vi "Update Speed.vi"(2 "error in (no error)":errorcluster, 3 "Time Since Last Update":dbl, 4 "Car.lvclass":refnum<class "Car.lvclass">) -> (0 "error out":errorcluster, 1 "Car.lvclass 2":refnum<class "Car.lvclass">)   [LabVIEW 2015, in "Car.lvclass"]
uses:
  Car.lvclass
  Car.lvclass/Car.ctl
panel:
  in  "Acceleration Rate":dbl=20.0
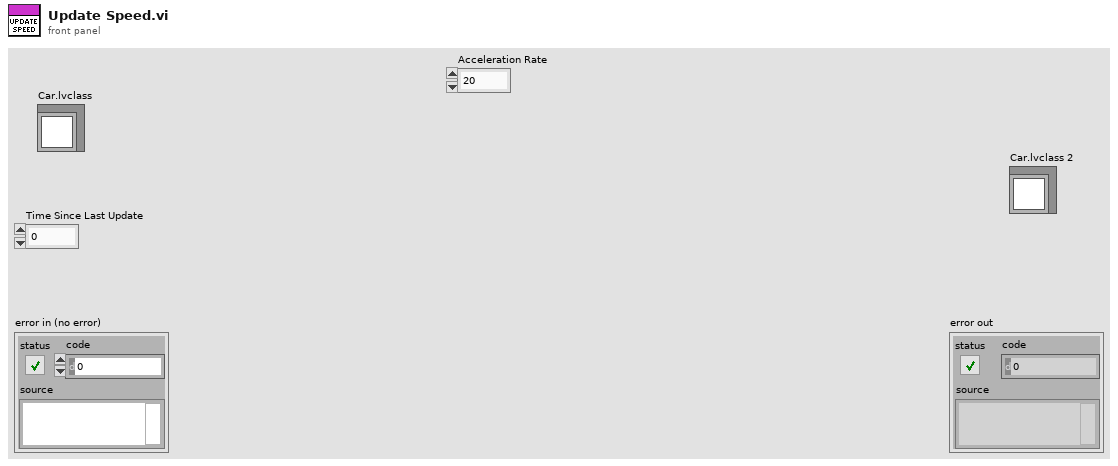
[diagram p1: front panel]
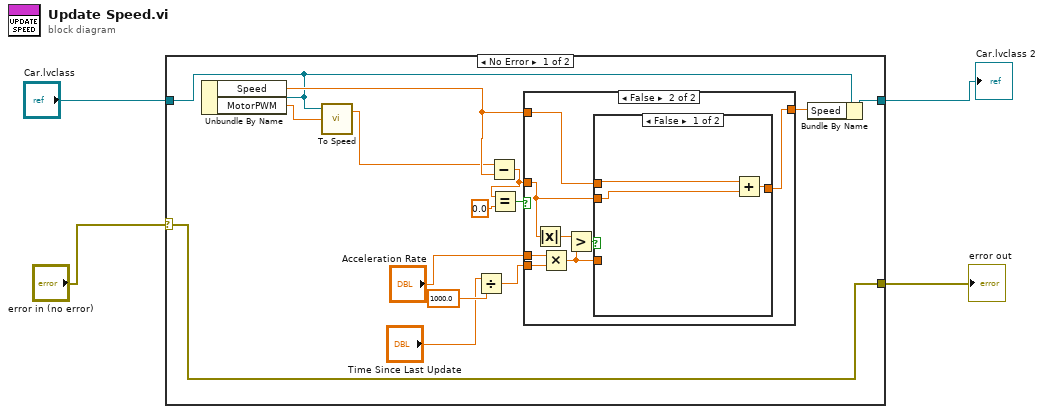
[diagram p0: block diagram]
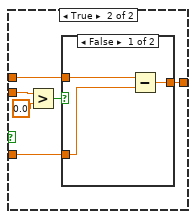
[diagram p3: hidden frame]
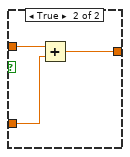
[diagram p4: hidden frame]
diagram:
  n1 = case shown="No Error" "error in (no error)" {
    selector: "error in (no error)" -> [w18 w44]
    tunnel: [w18 w44] -> w3
    tunnel: [w16 w43] -> w2
    tunnel: "Car.lvclass" -> [w6 w43]
    frame No Error {
      n2 = Unbundle By Name(w6) -> ("Speed"=w12:dbl, "MotorPWM"=w7:dbl)
      n3 = call "To Speed.vi"("Motor PWM"=w7, "Car.lvclass"=w6) -> ("Speed"=w5:dbl)  [unwired: 1 in, 1 out]
      n4 = Divide(x="Time Since Last Update", y=1000.0) -> (x/y=w8:dbl)
      n5 = Subtract(x=w5, y=w12) -> (x-y=w11:dbl)
      n6 = Equal?(x=w11, y=0.0) -> (x = y?=w15:bool)
      n7 = case shown="False" w15 {
        tunnel: "Acceleration Rate" -> [_ w27]
        tunnel: w8 -> [_ w26]
        tunnel: [w19 w20] -> w13
        tunnel: w12 -> [w19 w22]
        tunnel: w11 -> [_ w23]
        frame True {
        }
        frame False {
          n8 = Absolute Value(x=w23) -> (abs(x)=w24:dbl)
          n9 = Multiply(x=w27, y=w26) -> (x*y=w21:dbl)
          n10 = Greater?(x=w24, y=w21) -> (0:w25:bool)
          n11 = case shown="False" w25 {
            tunnel: w23 -> [w28 w35]
            tunnel: w22 -> [w29 w33]
            tunnel: w21 -> [_ w32]
            tunnel: [w30 w31] -> w20
            frame False {
              n12 = Add(x=w29, y=w28) -> (x+y=w30:dbl)
            }
            frame True {
              n13 = Greater?(x=w35, y=0.0) -> (0:w36:bool)
              n14 = case shown="False" w36 {
                tunnel: w33 -> [w38 w42]
                tunnel: w32 -> [w37 w41]
                tunnel: [w39 w40] -> w31
                frame False {
                  n15 = Subtract(x=w38, y=w37) -> (x-y=w39:dbl)
                }
                frame True {
                  n16 = Add(x=w42, y=w41) -> (x+y=w40:dbl)
                }
              }
            }
          }
        }
      }
      n17 = Bundle By Name(cluster=w6, "Speed"=w13) -> (w16:refnum<class "Car.lvclass">)
    }
    frame Error {
    }
  }
  "Car.lvclass 2" <- w2
  "error out" <- w3
